vi "Read File.vi"(8 "error in (no error)":errorcluster, 11 "Setup File in":refnum<class "Setup File.lvclass">) -> (0 "error out":errorcluster, 2 "Setup":T1, 3 "Setup File out":refnum<class "Setup File.lvclass">)   [LabVIEW 2018, in "Setup File.lvclass"]
doc: "Este VI faz a leitura do arquivo fornecido, escrevendo cada valor em formato string no cluster de saída \"Setup\"."
uses:
  Setup File.lvclass
  Setup File.lvclass/Setup File.ctl
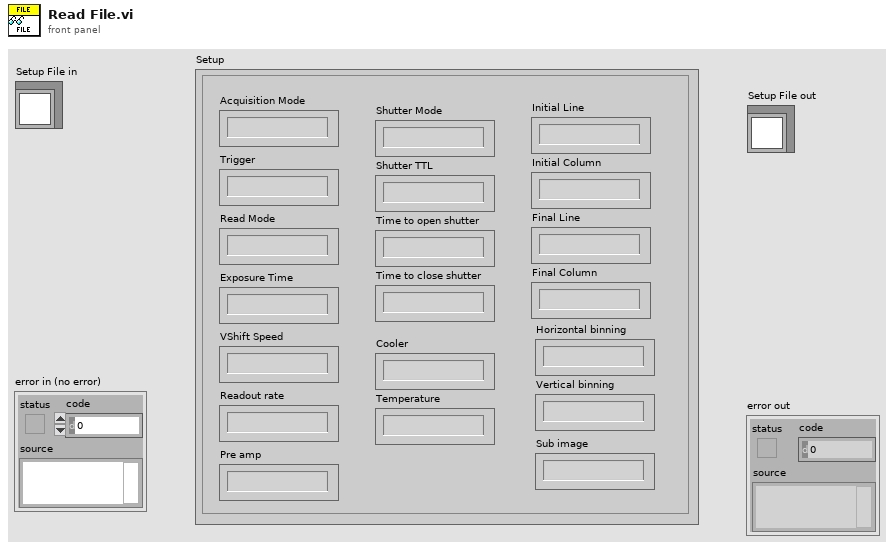
[diagram p1: front panel]
types:
  T1 = cluster{"Read Mode":string, "Acquisition Mode":string, "Trigger":string, "Exposure Time":string, "VShift Speed":string, "Readout rate":string, "Pre amp":string, "Shutter Mode":string, "Shutter TTL":string, "Time to open shutter":string, "Time to close shutter":string, "Cooler":string, "Temperature":string, "Initial Line":string, "Initial Column":string, "Final Line":string, "Final Column":string, "Horizontal binning":string, "Vertical binning":string, "Sub image":string}
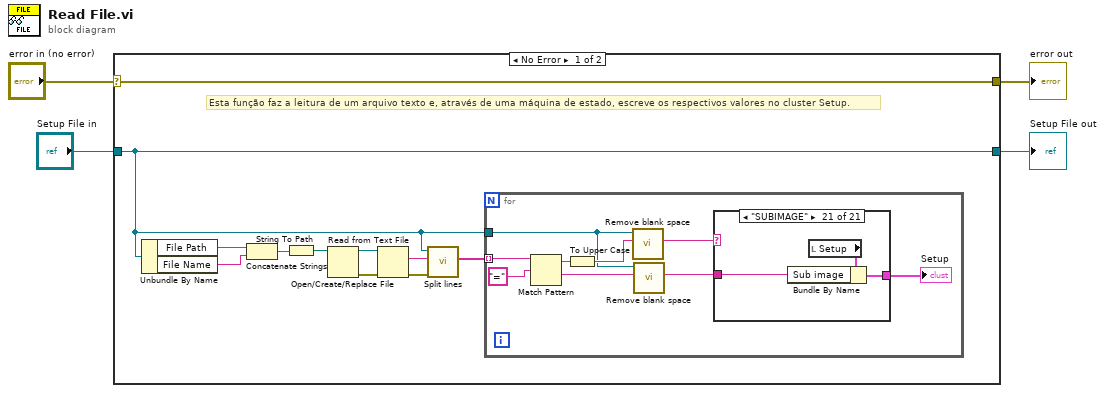
[diagram p0: block diagram]
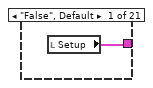
[diagram p2: hidden frame]
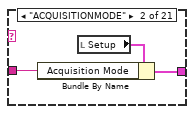
[diagram p3: hidden frame]
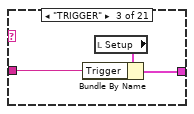
[diagram p4: hidden frame]
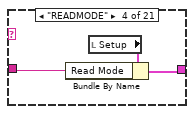
[diagram p5: hidden frame]
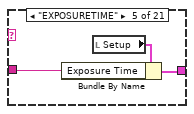
[diagram p6: hidden frame]
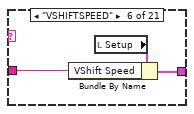
[diagram p7: hidden frame]
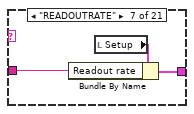
[diagram p8: hidden frame]
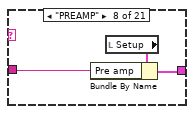
[diagram p9: hidden frame]
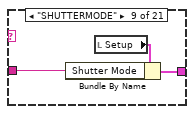
[diagram p10: hidden frame]
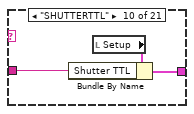
[diagram p11: hidden frame]
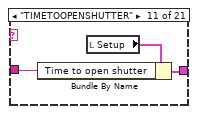
[diagram p12: hidden frame]
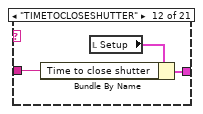
[diagram p13: hidden frame]
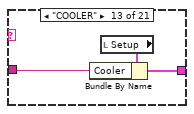
[diagram p14: hidden frame]
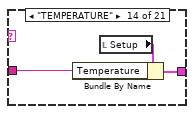
[diagram p15: hidden frame]
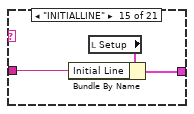
[diagram p16: hidden frame]
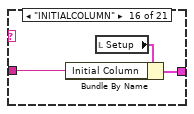
[diagram p17: hidden frame]
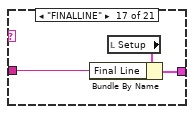
[diagram p18: hidden frame]
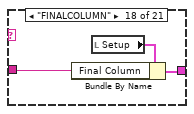
[diagram p19: hidden frame]
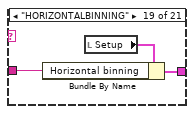
[diagram p20: hidden frame]
diagram:
  n1 = case shown="No Error" "error in (no error)" {
    selector: "error in (no error)" -> [w15 w86]
    tunnel: [w15 w86] -> w3
    tunnel: [w5 w87] -> w1
    tunnel: "Setup File in" -> [w5 w87]
    frame No Error {
      # "Esta função faz a leitura de um arquivo texto e, através de uma máquina de estado, escreve os respectivos valores no cluster Setup."
      n2 = Unbundle By Name(w5) -> ("File Path"=w11:string, "File Name"=w12:string)
      n3 = Concatenate Strings(w11, w12) -> (w10:string)
      n4 = String To Path(string=w10) -> (path=w9:path)
      n5 = Open/Create/Replace File(file path (use dialog)=w9) -> (refnum out=w13:refnum<file>, error out=w14:errorcluster)  [unwired: 5 in, 1 out]
      n6 = Read from Text File(file (use dialog)=w13, error in=w14) -> (text=w7:string, error out=w8:errorcluster)  [unwired: 2 in, 2 out]
      n7 = call "Split lines.vi"("error in (no error)"=w8, "spreadsheet string"=w7, "Setup File in"=w5) -> ("array"=w6:string[])  [unwired: 6 in, 2 out]
      n8 = for {
        tunnel: w6 -> [w24] mode=indexing
        tunnel: w5 -> [w16]
        n9 = Match Pattern(string=w24, regular expression="=" ("search string/char (-)")) -> (before substring=w22:string, after substring=w21:string)  [unwired: 1 in, 2 out]
        n10 = To Upper Case(1:w22) -> (0:w18:string)
        n11 = call "Remove blank space.vi"("string in"=w18, "Setup File in"=w16) -> ("string out"=w17:string)  [unwired: 7 in, 2 out]
        n12 = call "Remove blank space.vi"("string in"=w21, "Setup File in"=w16) -> ("string out"=w20:string)  [unwired: 7 in, 2 out]
        n13 = case shown="\"SUBIMAGE\"" w17 {
          tunnel: w20 -> [_ w26 w30 w33 w35 w38 w41 w44 w47 w50 w53 w56 w60 w63 w65 w68 w71 w74 w77 w80 w84]
          tunnel: [w25 w27 w29 w32 w36 w39 w42 w45 w48 w51 w54 w57 w59 w62 w66 w69 w72 w75 w78 w81 w83] -> w19
          frame "False", Default {
            n14 = local read "Setup"() -> (w25:T1)
          }
          frame "ACQUISITIONMODE" {
            n15 = local read "Setup"() -> (w28:T1)
            n16 = Bundle By Name(cluster=w28, "Acquisition Mode"=w26) -> (w27:T1)
          }
          frame "TRIGGER" {
            n17 = local read "Setup"() -> (w31:T1)
            n18 = Bundle By Name(cluster=w31, "Trigger"=w30) -> (w29:T1)
          }
          frame "READMODE" {
            n19 = local read "Setup"() -> (w34:T1)
            n20 = Bundle By Name(cluster=w34, "Read Mode"=w33) -> (w32:T1)
          }
          frame "EXPOSURETIME" {
            n21 = local read "Setup"() -> (w37:T1)
            n22 = Bundle By Name(cluster=w37, "Exposure Time"=w35) -> (w36:T1)
          }
          frame "VSHIFTSPEED" {
            n23 = local read "Setup"() -> (w40:T1)
            n24 = Bundle By Name(cluster=w40, "VShift Speed"=w38) -> (w39:T1)
          }
          frame "READOUTRATE" {
            n25 = local read "Setup"() -> (w43:T1)
            n26 = Bundle By Name(cluster=w43, "Readout rate"=w41) -> (w42:T1)
          }
          frame "PREAMP" {
            n27 = local read "Setup"() -> (w46:T1)
            n28 = Bundle By Name(cluster=w46, "Pre amp"=w44) -> (w45:T1)
          }
          frame "SHUTTERMODE" {
            n29 = local read "Setup"() -> (w49:T1)
            n30 = Bundle By Name(cluster=w49, "Shutter Mode"=w47) -> (w48:T1)
          }
          frame "SHUTTERTTL" {
            n31 = local read "Setup"() -> (w52:T1)
            n32 = Bundle By Name(cluster=w52, "Shutter TTL"=w50) -> (w51:T1)
          }
          frame "TIMETOOPENSHUTTER" {
            n33 = local read "Setup"() -> (w55:T1)
            n34 = Bundle By Name(cluster=w55, "Time to open shutter"=w53) -> (w54:T1)
          }
          frame "TIMETOCLOSESHUTTER" {
            n35 = local read "Setup"() -> (w58:T1)
            n36 = Bundle By Name(cluster=w58, "Time to close shutter"=w56) -> (w57:T1)
          }
          frame "COOLER" {
            n37 = local read "Setup"() -> (w61:T1)
            n38 = Bundle By Name(cluster=w61, "Cooler"=w60) -> (w59:T1)
          }
          frame "TEMPERATURE" {
            n39 = local read "Setup"() -> (w64:T1)
            n40 = Bundle By Name(cluster=w64, "Temperature"=w63) -> (w62:T1)
          }
          frame "INITIALLINE" {
            n41 = local read "Setup"() -> (w67:T1)
            n42 = Bundle By Name(cluster=w67, "Initial Line"=w65) -> (w66:T1)
          }
          frame "INITIALCOLUMN" {
            n43 = local read "Setup"() -> (w70:T1)
            n44 = Bundle By Name(cluster=w70, "Initial Column"=w68) -> (w69:T1)
          }
          frame "FINALLINE" {
            n45 = local read "Setup"() -> (w73:T1)
            n46 = Bundle By Name(cluster=w73, "Final Line"=w71) -> (w72:T1)
          }
          frame "FINALCOLUMN" {
            n47 = local read "Setup"() -> (w76:T1)
            n48 = Bundle By Name(cluster=w76, "Final Column"=w74) -> (w75:T1)
          }
          frame "HORIZONTALBINNING" {
            n49 = local read "Setup"() -> (w79:T1)
            n50 = Bundle By Name(cluster=w79, "Horizontal binning"=w77) -> (w78:T1)
          }
          frame "VERTICALBINNING" {
            n51 = local read "Setup"() -> (w82:T1)
            n52 = Bundle By Name(cluster=w82, "Vertical binning"=w80) -> (w81:T1)
          }
          frame "SUBIMAGE" {
            n53 = local read "Setup"() -> (w85:T1)
            n54 = Bundle By Name(cluster=w85, "Sub image"=w84) -> (w83:T1)
          }
        }
        "Setup" <- w19
      }
    }
    frame Error {
    }
  }
  "error out" <- w3
  "Setup File out" <- w1
